vi "shutter-user-event-out-global.vi"() -> ()   [LabVIEW 2014]
uses:
  user event shutter global.ctl
panel:
  in  "user event":refnum<user-event>
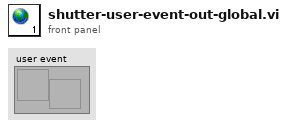
[diagram p1: front panel]
diagram:
